vi "Get_card_parameters_from_user.vi"(4 "External Trigger?":bool=TRUE, 6 "Trigger Level":i32(slide)=29 min=-100 max=100 step=1 scale=-100.0..100.0, 8 "error in (no error)":errorcluster, 9 "Range":u32(ring)=10000 items=["+/- 5 V"=10000, "+/- 2 V"=4000, "+/- 1 V"=2000, "+/- 500 mV"=1000, "+/- 200 mV"=400, "+/- 100 mV"=200], 10 "Number of points":dbl=816000.0, 11 "Control_interface in":refnum<class "Control_interface.lvclass">) -> (0 "error out":errorcluster, 3 "Control_interface out":refnum<class "Control_interface.lvclass">)   [LabVIEW 2015, in "Control_interface.lvclass"]
uses:
  Control_interface.lvclass
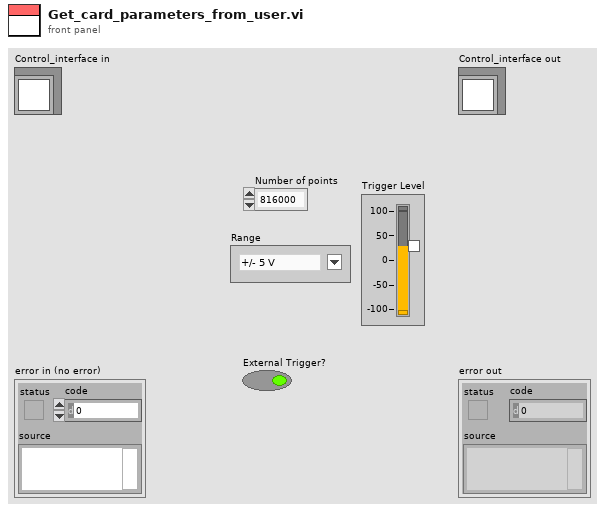
[diagram p1: front panel]
types:
  T1 = cluster{"Sample Rate":dbl, "Clock mode":enum16{"Internal", "External", "Reference"}, "Mode":u16, "Depth":dbl, "Segment Size":dbl, "Trigger Timeout":dbl, "Trigger Holdoff":dbl, "Trigger Delay":dbl}
  T2 = cluster{"Coupling":u16, "Differential Input":bool, "Direct-to-ADC":bool, "Range":u32, "Impedance":u32, "DC Offset":i32, "Filter":i32}
  T3 = cluster{"Slope":u16, "Level":i32, "Source":i32, "External Range":u32, "External Coupling":u16, "External":bool, "Disable":bool, "External Impedance":u16}
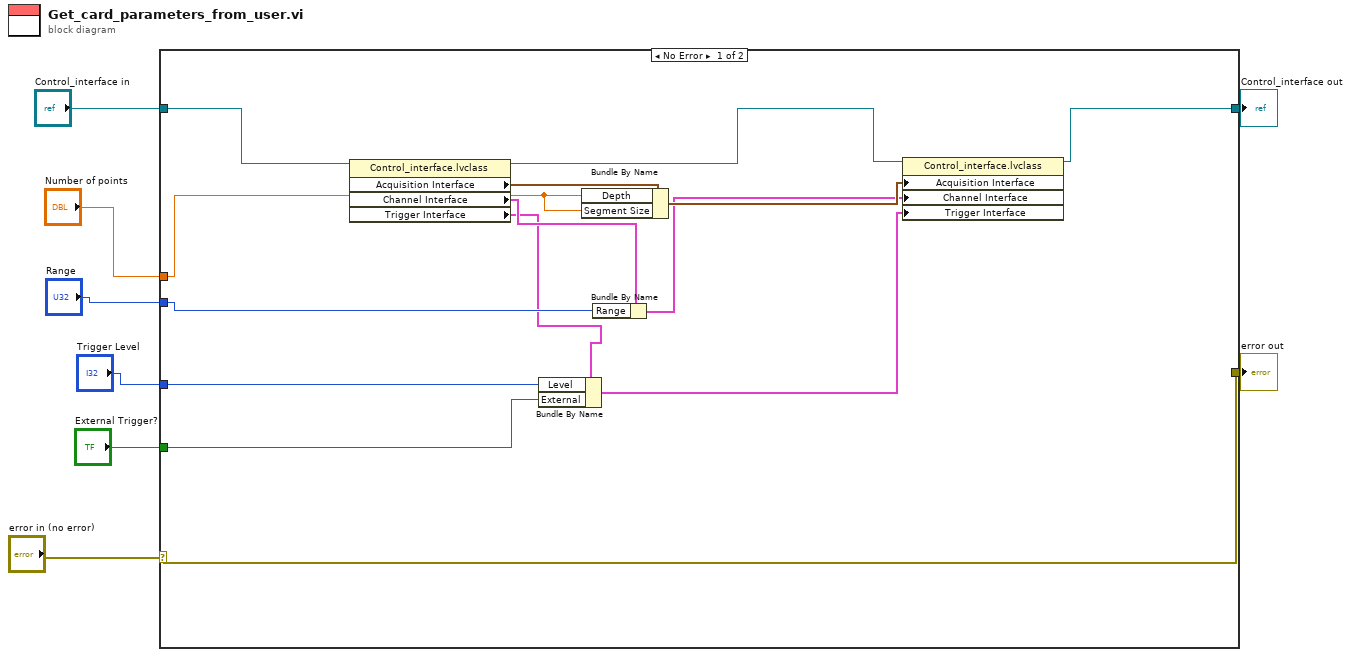
[diagram p0: block diagram]
diagram:
  n1 = case shown="No Error" "error in (no error)" {
    selector: "error in (no error)" -> [w22 w24]
    tunnel: [w22 w24] -> w7
    tunnel: [w18 w23] -> w5
    tunnel: "Control_interface in" -> [w21 w23]
    tunnel: "Number of points" -> [w17 _]
    tunnel: "Range" -> [w13 _]
    tunnel: "Trigger Level" -> [w10 _]
    tunnel: "External Trigger?" -> [w9 _]
    frame No Error {
      n2 = property class="Control_interface.lvclass"(reference=w21) -> (reference out=w19:refnum<class "Control_interface.lvclass">, "Acquisition Interface"=w20:T1, "Channel Interface"=w15:T2, "Trigger Interface"=w12:T3)  [unwired: 1 in, 1 out]
      n3 = Bundle By Name(cluster=w12, "Level"=w10, "External"=w9) -> (w11:T3)
      n4 = Bundle By Name(cluster=w20, "Depth"=w17, "Segment Size"=w17) -> (w16:T1)
      n5 = Bundle By Name(cluster=w15, "Range"=w13) -> (w14:T2)
      n6 = property class="Control_interface.lvclass"(reference=w19, "Acquisition Interface"=w16, "Channel Interface"=w14, "Trigger Interface"=w11) -> (reference out=w18:refnum<class "Control_interface.lvclass">)  [unwired: 1 in, 1 out]
    }
    frame Error {
    }
  }
  "error out" <- w7
  "Control_interface out" <- w5
